vi "数组函数的使用.vi"() -> ()   [LabVIEW 2018]
panel:
  out "移动后的新的数组":dbl[][](array[numeric])
  out "反转数组":dbl[][](array[numeric])
  out "原始数组":dbl[][](array[numeric])
  # "创建一个VI，产生一个4行6列的数组，数组内数值范围为1-100内的整数，\n显示该数组后（原始数组），再将数组的每行元素颠倒过来，生成新数组\n进行显示，最后再将原始组数的前3个元素移到数组最后端，形成新的数\n组显示出来。"
  # "20174080221\n王靖\n电子二班"
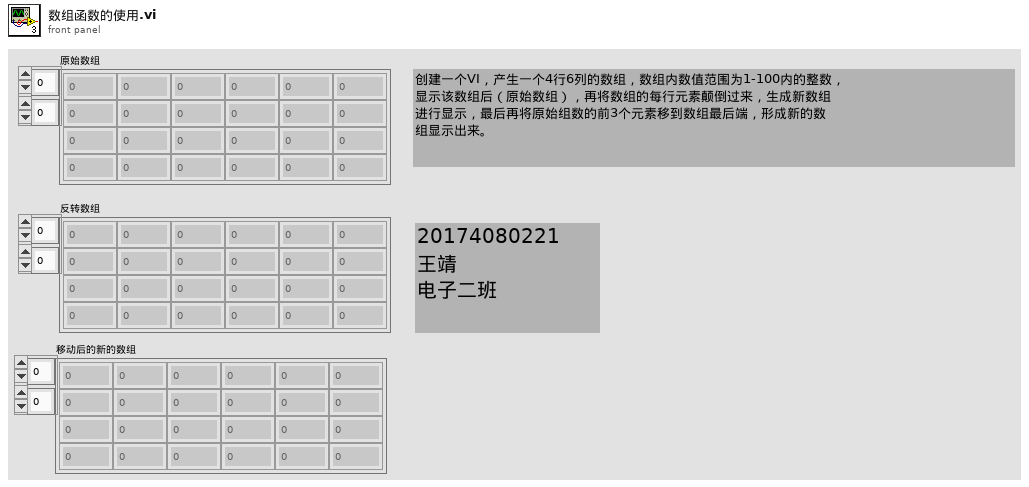
[diagram p1: front panel]
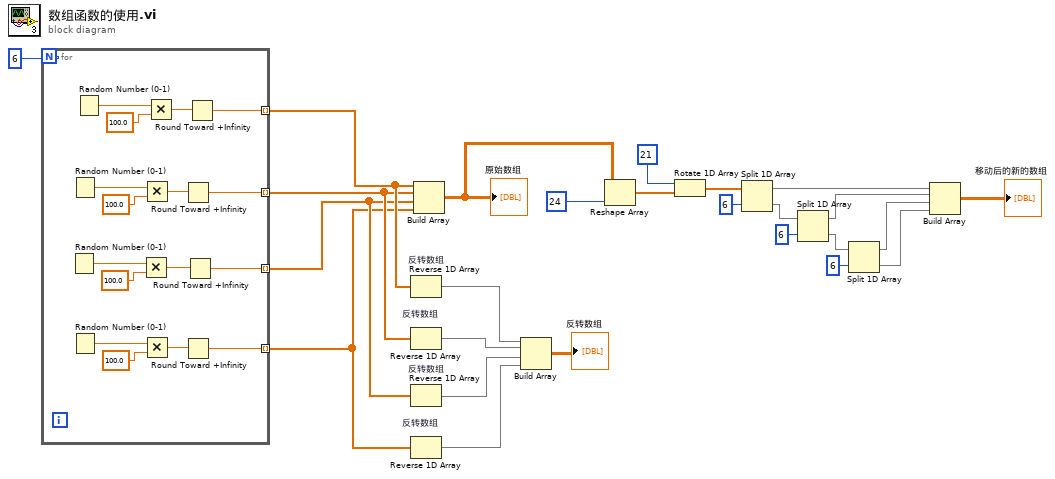
[diagram p0: block diagram]
diagram:
  n1 = for {
    N: 6 -> [_]
    tunnel: [w29] -> w24 mode=indexing
    tunnel: [w28] -> w23 mode=indexing
    tunnel: [w27] -> w22 mode=indexing
    tunnel: [w26] -> w21 mode=indexing
    n2 = Random Number (0-1)() -> (number: 0 to 1=w35:dbl)
    n3 = Random Number (0-1)() -> (number: 0 to 1=w38:dbl)
    n4 = Random Number (0-1)() -> (number: 0 to 1=w32:dbl)
    n5 = Random Number (0-1)() -> (number: 0 to 1=w41:dbl)
    n6 = Multiply(x=w35, y=100.0) -> (x*y=w33:dbl)
    n7 = Multiply(x=w38, y=100.0) -> (x*y=w36:dbl)
    n8 = Multiply(x=w32, y=100.0) -> (x*y=w30:dbl)
    n9 = Multiply(x=w41, y=100.0) -> (x*y=w39:dbl)
    n10 = Round Toward +Infinity(x=w36) -> (ceil(x): smallest int >= x=w28:dbl)
    n11 = Round Toward +Infinity(x=w30) -> (ceil(x): smallest int >= x=w26:dbl)
    n12 = Round Toward +Infinity(x=w33) -> (ceil(x): smallest int >= x=w27:dbl)
    n13 = Round Toward +Infinity(x=w39) -> (ceil(x): smallest int >= x=w29:dbl)
  }
  n14 = Reverse 1D Array "反转数组"(array=w24) -> (reversed array=w20:dbl[])
  n15 = Reverse 1D Array "反转数组"(array=w23) -> (reversed array=w19:dbl[])
  n16 = Reverse 1D Array "反转数组"(array=w22) -> (reversed array=w18:dbl[])
  n17 = Reverse 1D Array "反转数组"(array=w21) -> (reversed array=w17:dbl[])
  n18 = Build Array(w24, w23, w22, w21) -> (w15:dbl[][])
  "原始数组" <- w15
  n19 = Build Array(w20, w19, w18, w17) -> (→"反转数组":dbl[][])
  n20 = Reshape Array(w15, 24 ("维数大小")) -> (w12:dbl[])
  n21 = Rotate 1D Array(1:w12, 2:21 ("n")) -> (0:w11:dbl[])
  n22 = Split 1D Array(array=w11, index=6 ("索引")) -> (first subarray=w5:dbl[], second subarray=w7:dbl[])
  n23 = Split 1D Array(array=w7, index=6 ("索引")) -> (first subarray=w4:dbl[], second subarray=w6:dbl[])
  n24 = Split 1D Array(array=w6, index=6 ("索引")) -> (first subarray=w3:dbl[], second subarray=w2:dbl[])
  n25 = Build Array(w5, w4, w3, w2) -> (→"移动后的新的数组":dbl[][])
